vi "ConfigParams - Parse - OperationalModes.vi"(8 "error in (no error)":errorcluster, 11 "Ethernet in":refnum<class "ENET_BS1201.lvclass">) -> (0 "error out":errorcluster, 2 "CellInhibitEnable":bool, 3 "Ethernet out":refnum<class "ENET_BS1201.lvclass">)   [LabVIEW 2021, in "BS120x Driver.lvlib" / "ENET_BS1201.lvclass"]
doc: "Configure the Cell Inhibit Enable function. Unit must be restarted to take effect."
uses:
  ENET_BS1201.lvclass
  ENET_BS1201.lvclass/ENET_BS1201.ctl
panel:
  # "[OperationalModes]\nCellInhibitEnable = False"
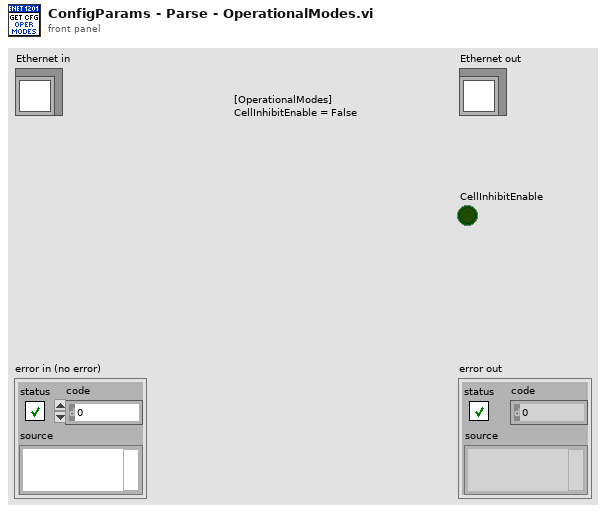
[diagram p1: front panel]
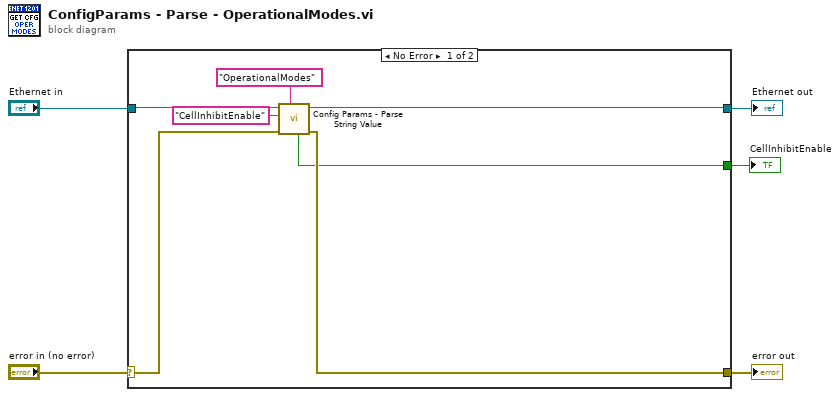
[diagram p0: block diagram]
diagram:
  n1 = case shown="No Error" "error in (no error)" {
    selector: "error in (no error)" -> [w9 w14]
    tunnel: [w7 w14] -> w4
    tunnel: [w8 w13] -> w2
    tunnel: "Ethernet in" -> [w12 w13]
    tunnel: [w6 _] -> w1
    frame No Error {
      n2 = call-dynamic "Config Params - Parse String Value.vi"("Section"="OperationalModes", "error in (no error)"=w9, "Key"="CellInhibitEnable", "Ethernet in"=w12) -> ("error out"=w7:errorcluster, "Ethernet out"=w8:refnum<class "ENET_BS1201.lvclass">, "Value (bool)"=w6:bool)  [unwired: 1 in, 4 out]
    }
    frame Error {
    }
  }
  "error out" <- w4
  "Ethernet out" <- w2
  "CellInhibitEnable" <- w1
